vi "Register Plugin.vi"(6 "Version":T1, 8 "error in (no error)":errorcluster, 9 "gRPC Port":i32, 10 "Unique Name":string, 11 "Launcher in":refnum<class "CIFPluginManager.lvclass">) -> (0 "error out":errorcluster, 3 "Launcher out":refnum<class "CIFPluginManager.lvclass">)   [LabVIEW 2021, in "CIFPluginManager.lvclass"]
uses:
  CIFPluginManager.lvclass
  CIFCore/Common/Typedef/Version.ctl
  CIFPluginManager.lvclass/CIFPluginManager.ctl
  <vilib>/Utility/miscctls.llb/LVMapReplaceAction.ctl
  CIFCore/Common/Typedef/Errors.ctl
  <vilib>/CIF Foundation/CIF Utilities/Errors/Append Error Location.vi
  CIFCore/Common/CIFCoreCommon.lvlib
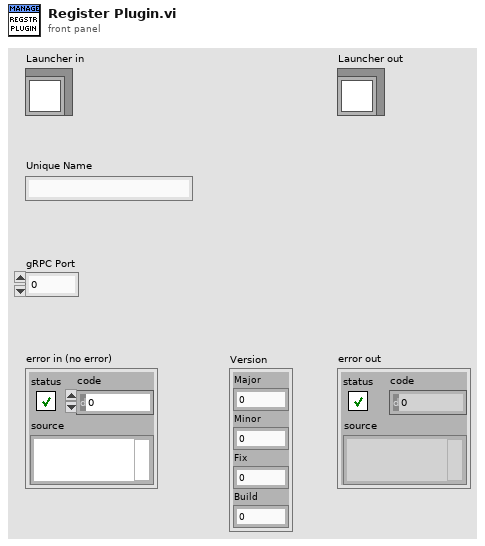
[diagram p1: front panel]
types:
  T1 = typedef "CIFCoreCommon.lvlib/Version.ctl" = cluster{"Major":i32, "Minor":i32, "Fix":i32, "Build":i32}
  T2 = typedef "LVMapReplaceAction.ctl" = enum32{"Modify Entry only if found", "Add or Modify Entry", "Delete Entry"}
  T3 = typedef "CIFCoreCommon.lvlib/Errors.ctl" = enum16{"Invalid Clock ID", "Long Sleep", "gRPC Server Not Found", "Config Parse", "Timestamp Wrap", "Delayed Execution", "Duplicate Channel", "Missing Channel", "Incorrect Type", "Flatten Error", "Unflatten Data", "Unique Name", "Plugin Not Found", "Plugin Type Not Found", "Plugin Version Not Found", "Manager Not Found", "Numerical Issue", "Time Jump", "Clock ID Match", "Channel Length", "Plugin Connection", "gRPC Server Connection", "PPL Name Match", "Build", "Config Log Parse", "Plugin Load", "UI Subpanel Load", "Python Name", "Invalid Name"}
  T4 = typedef "CIFPluginManager.lvclass/Plugin Management Data.ctl" = cluster{"vi reference":refnum<vi>, "gRPC ID":T5, "Plugin Type":string, "Unique Name":string, "gRPC Port":i32, "Version":T1, "Load Timestamp":i64, "Unload Timestamp":i64, "Unloading":bool, "Ready for removal":bool, "status":T6}
  T5 = typedef "grpc-lvsupport-release.lvlib/grpcId.ctl" = u64
  T6 = typedef "CIF_Manager_server.lvlib/cif_plugincore_StatusData.ctl" = cluster{"state":T7, "timing_statistics":T8, "fifo_statistics":T10, "error":T11, "monitor_doubles":T12, "monitor_u64s":T13, "monitor_i64s":T14}
  T7 = typedef "CIF_Manager_server.lvlib/cif_plugincore_StatusData_State.ctl" = enum32{"NULL", "CREATING", "LISTENING", "RUNNING", "CLEANINGUP", "DESTROYING"}
  T8 = typedef "CIF_Manager_server.lvlib/cif_plugincore_TimingStatistics.ctl" = cluster{"period":T9, "wake_error":T9, "execute":T9, "housekeep":T9, "idle":T9, "cleanup":T9, "custom_1":T9, "custom_2":T9}
  T9 = typedef "CIF_Manager_server.lvlib/cif_common_TimingStats.ctl" = cluster{"max":i64, "min":i64, "avg":dbl}
  T10 = typedef "CIF_Manager_server.lvlib/cif_plugincore_FifoStatistics.ctl" = cluster{"from_t0":T9, "from_previous_plugin":T9, "output_error":T9}
  T11 = typedef "CIF_Manager_server.lvlib/cif_plugincore_Error.ctl" = cluster{"status":bool, "code":i32}
  T12 = typedef "CIF_Manager_server.lvlib/cif_plugincore_MonitorDoubles.ctl" = cluster{"double_1":dbl, "double_2":dbl, "double_3":dbl, "double_4":dbl}
  T13 = typedef "CIF_Manager_server.lvlib/cif_plugincore_MonitorU64.ctl" = cluster{"u64_1":u64, "u64_2":u64, "u64_3":u64, "u64_4":u64}
  T14 = typedef "CIF_Manager_server.lvlib/cif_plugincore_MonitorI64.ctl" = cluster{"i64_1":i64, "i64_2":i64, "i64_3":i64, "i64_4":i64}
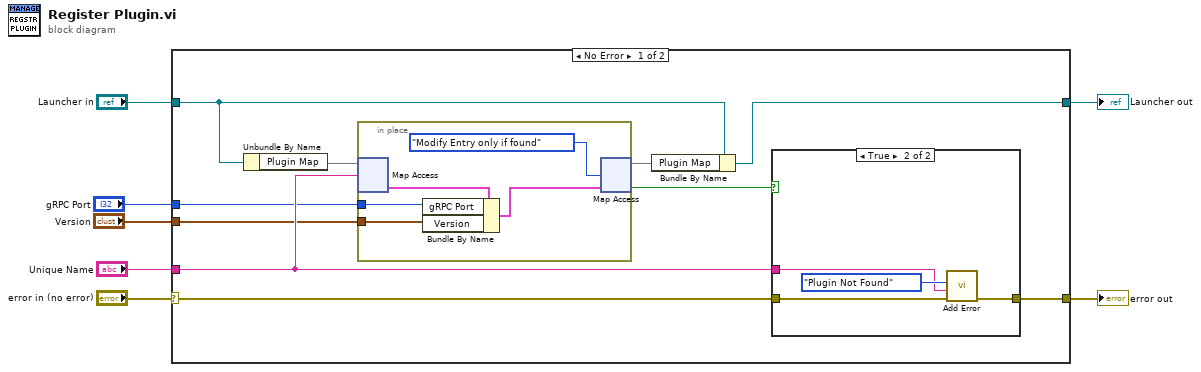
[diagram p0: block diagram]
diagram:
  n1 = case shown="No Error" "error in (no error)" {
    selector: "error in (no error)" -> [w17 w29]
    tunnel: [w16 w29] -> w6
    tunnel: [w8 w28] -> w4
    tunnel: "Launcher in" -> [w11 w28]
    tunnel: "Unique Name" -> [w14 _]
    tunnel: "Version" -> [w13 _]
    tunnel: "gRPC Port" -> [w12 _]
    frame No Error {
      n2 = Unbundle By Name(w11) -> ("Plugin Map"=w15:map{string, T4})
      n3 = in-place {
        in-place-border: w13 -> [w20]
        in-place-border: w12 -> [w19]
        n4 = in-place-map #1(w15, w14) -> (w21:T4)  [unwired: 1 in, 1 out]
        n5 = Bundle By Name(cluster=w21, "gRPC Port"=w19, "Version"=w20) -> (w18:T4)
        n6 = in-place-map #1(w18, LVMapReplaceAction."Modify Entry only if found" ("action")) -> (w10:map{string, T4}, w9:bool)  [unwired: 1 out]
      }
      n7 = Bundle By Name(cluster=w11, "Plugin Map"=w10) -> (w8:refnum<class "CIFPluginManager.lvclass">)
      n8 = case shown="True" w9 {
        tunnel: w17 -> [w23 w27]
        tunnel: [w23 w24] -> w16
        tunnel: w14 -> [_ w25]
        frame False {
        }
        frame True {
          n9 = call "Add Error.vi"("error in (no error)"=w27, "String to Append"=w25, "Error"=Errors."Plugin Not Found") -> ("error out"=w24:errorcluster)  [unwired: 8 in]
        }
      }
    }
    frame Error {
    }
  }
  "error out" <- w6
  "Launcher out" <- w4
